vi "set_velocity.vi"(8 "error in (no error)":errorcluster, 10 "Velocity (steps/sec)":i32, 11 "Picomotor in":refnum<class "Picomotor.lvclass">) -> (0 "error out":errorcluster, 3 "Picomotor out":refnum<class "Picomotor.lvclass">)   [LabVIEW 2020, in "Picomotor.lvclass"]
uses:
  Picomotor.lvclass
  Picomotor.lvclass/Picomotor.ctl
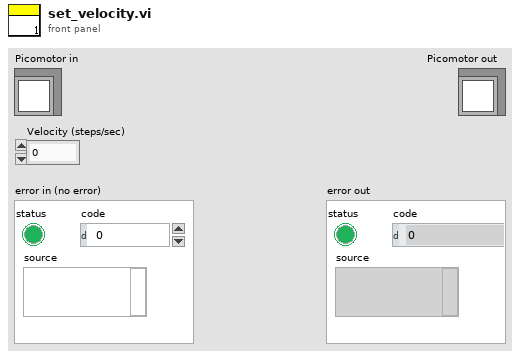
[diagram p1: front panel]
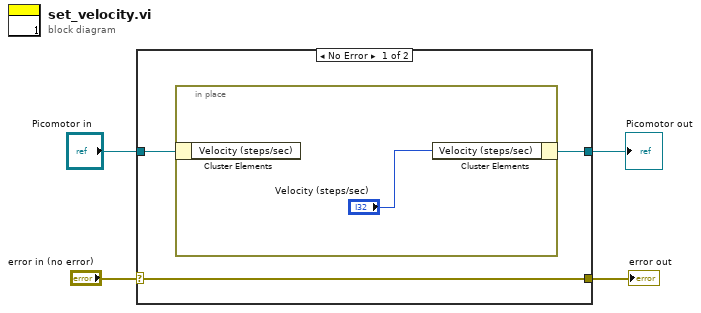
[diagram p0: block diagram]
diagram:
  n1 = case shown="No Error" "error in (no error)" {
    selector: "error in (no error)" -> [w7 w10]
    tunnel: [w7 w10] -> w3
    tunnel: [w5 w9] -> w1
    tunnel: "Picomotor in" -> [w6 w9]
    frame No Error {
      n2 = in-place {
        n3 = in-place-cluster #1(w6) -> ()  [unwired: 1 out]
        n4 = in-place-cluster #1("Velocity (steps/sec)"="Velocity (steps/sec)") -> (w5:refnum<class "Picomotor.lvclass">)
      }
    }
    frame Error {
    }
  }
  "error out" <- w3
  "Picomotor out" <- w1
